vi "SetPositionUm.vi"(8 "error in (no error)":errorcluster, 9 "Positionum":dbl min=0.0 max=200.0, 10 "Stage Label":string, 11 "Stage_MadCityLab in":refnum<class "Stage_MadCityLab.lvclass">) -> (0 "error out":errorcluster, 3 "Stage_MadCityLab out":refnum<class "Stage_MadCityLab.lvclass">)   [LabVIEW 2020, in "Stage_MadCityLab.lvlib" / "Stage_MadCityLab.lvclass"]
uses:
  Stage_MadCityLab.lvclass
  Stage_MadCityLab.lvclass/Stage_MadCityLab.ctl
  HAL Layer/Stage/Stage/Stage.lvclass
  Dependency/Madlib.dll
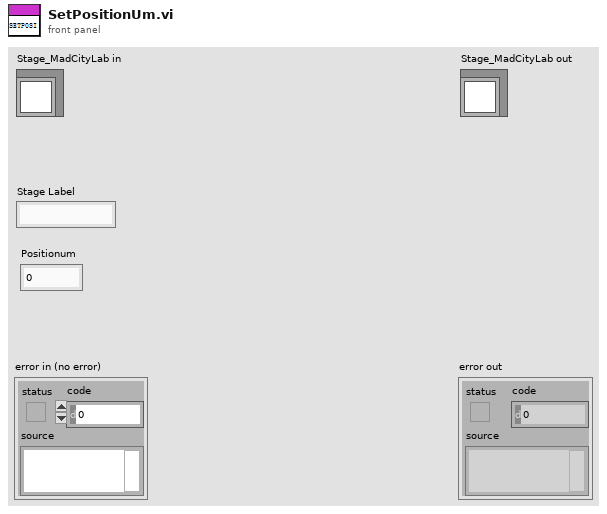
[diagram p1: front panel]
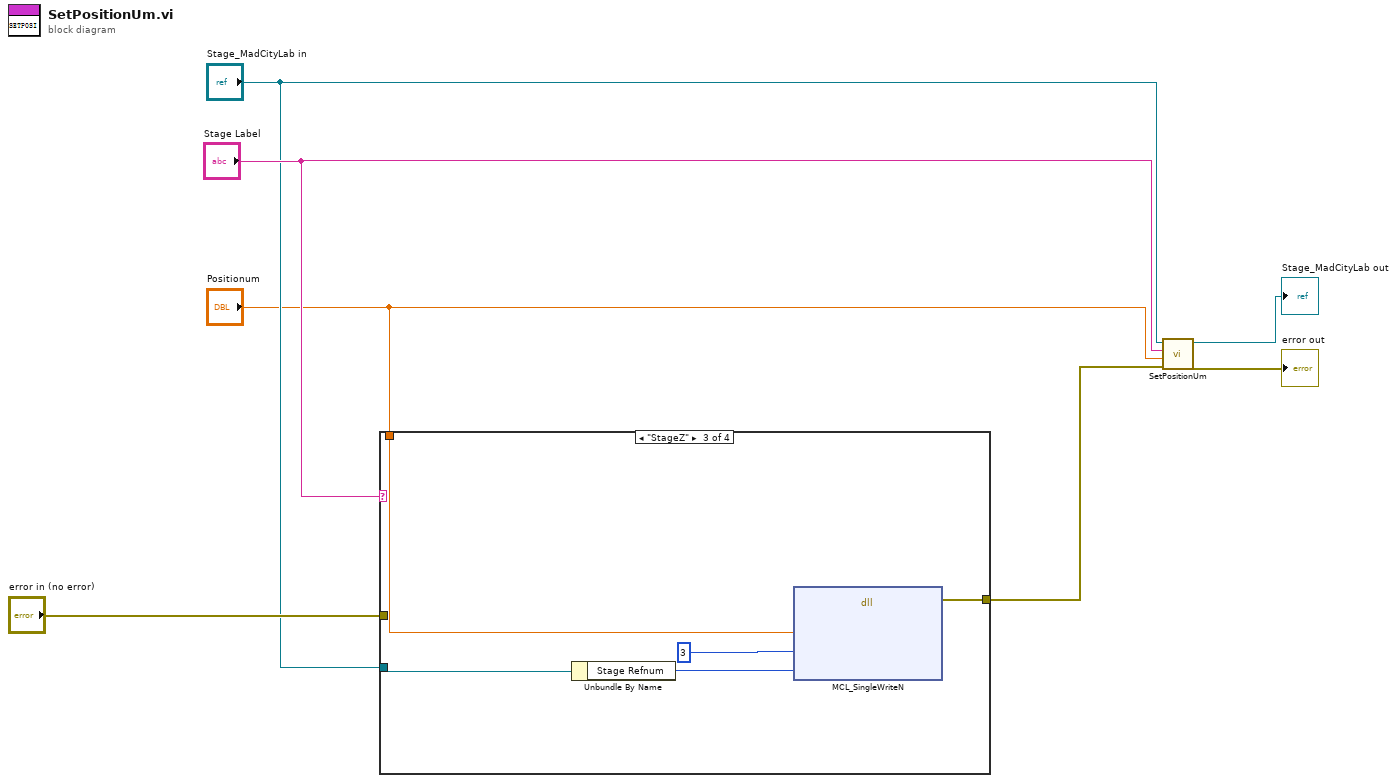
[diagram p0: block diagram]
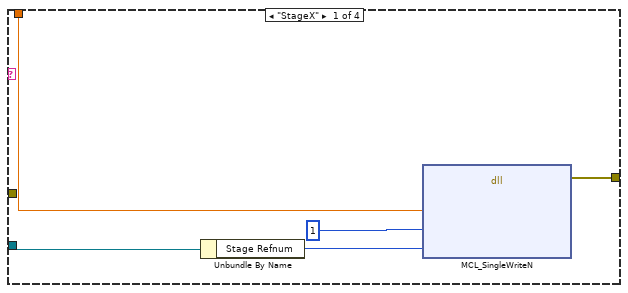
[diagram p2: hidden frame]
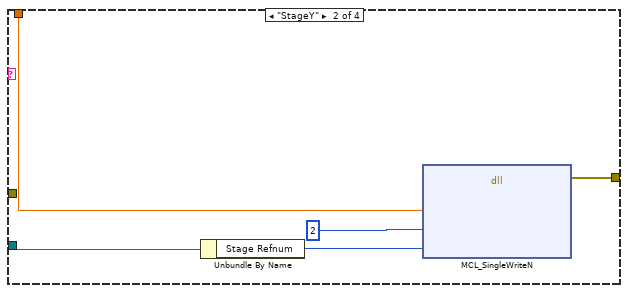
[diagram p3: hidden frame]
diagram:
  n1 = case shown="\"StageZ\"" "Stage Label" {
    tunnel: [w12 w17 w22 w23] -> w3
    tunnel: "error in (no error)" -> [_ _ _ w23]
    tunnel: "Stage_MadCityLab in" -> [w11 w16 w21 _]
    tunnel: "Positionum" -> [w8 w13 w18 _]
    frame "StageX" {
      n2 = Unbundle By Name(w11) -> ("Stage Refnum"=w10:i32)
      n3 = dll-call lib="E:/Development/DevHardSoftware/MMicroscopyAF/Model/Real Hardware/Stage_MadCityLab/Stage_MadCityLab/Dependency/Madlib.dll" fn="MCL_SingleWriteN"("position"=w8, "axis"=u32 1, "handle"=w10) -> (error out=w12:errorcluster)  [unwired: 7 in, 1 out]
    }
    frame "StageY" {
      n4 = Unbundle By Name(w16) -> ("Stage Refnum"=w15:i32)
      n5 = dll-call lib="E:/Development/DevHardSoftware/MMicroscopyAF/Model/Real Hardware/Stage_MadCityLab/Stage_MadCityLab/Dependency/Madlib.dll" fn="MCL_SingleWriteN"("position"=w13, "axis"=u32 2, "handle"=w15) -> (error out=w17:errorcluster)  [unwired: 7 in, 1 out]
    }
    frame "StageZ" {
      n6 = Unbundle By Name(w21) -> ("Stage Refnum"=w20:i32)
      n7 = dll-call lib="E:/Development/DevHardSoftware/MMicroscopyAF/Model/Real Hardware/Stage_MadCityLab/Stage_MadCityLab/Dependency/Madlib.dll" fn="MCL_SingleWriteN"("position"=w18, "axis"=u32 3, "handle"=w20) -> (error out=w22:errorcluster)  [unwired: 7 in, 1 out]
    }
    frame Default {
    }
  }
  n8 = call-parent "SetPositionUm.vi"("error in (no error)"=w3, "Positionum"="Positionum", "Stage Label"="Stage Label", "Stage in"="Stage_MadCityLab in") -> ("error out"=→"error out":errorcluster, "Stage out"=→"Stage_MadCityLab out":refnum<class "Stage_MadCityLab.lvclass">)  [unwired: 6 in]
